vi "Initialize Menu Panel.vi"(8 "error in":errorcluster, 11 "Display State In":T1={"Numeric"=0.0, "Array of Button References"=[], "Space Between Menu Buttons"=0, "Number of Menu Buttons"=0, "Array of Button Names"=[], "Most Recent Vertical Position"=0, "This VI"=refnum, "Current Action"=enum."Not Moving", "Most Recent Distance Traveled"=0, "Method"=enum."Move Up", "Data In"=0}) -> (0 "error IO 2":errorcluster, 3 "Display State Out":T1={"Numeric"=0.0, "Array of Button References"=[], "Space Between Menu Buttons"=3, "Number of Menu Buttons"=6, "Array of Button Names"=[], "Most Recent Vertical Position"=0, "This VI"=refnum, "Current Action"=enum."Not Moving", "Most Recent Distance Traveled"=0, "Method"=enum."Resize", "Data In"=0} caption="State")   [LabVIEW 2011, in "Sliding Menu Library.lvlib" / "Sliding Menu XControl.xctl"]
uses:
  Sliding Menu xControl/Sliding Menu XControl.xctl
  Sliding Menu xControl/Sliding Menu State.ctl
  Menu Button Library/Menu Button xControl/Menu Button xControl.xctl
  Sliding Menu Type Definitions/Current User Action.ctl
  Sliding Menu xControl/Sliding Menu Methods.ctl
  Sliding Menu xControl/Sliding Menu Data.ctl
  <vilib>/Utility/miscctls.llb/LVPointTypeDef.ctl
  Sliding Menu Library.lvlib
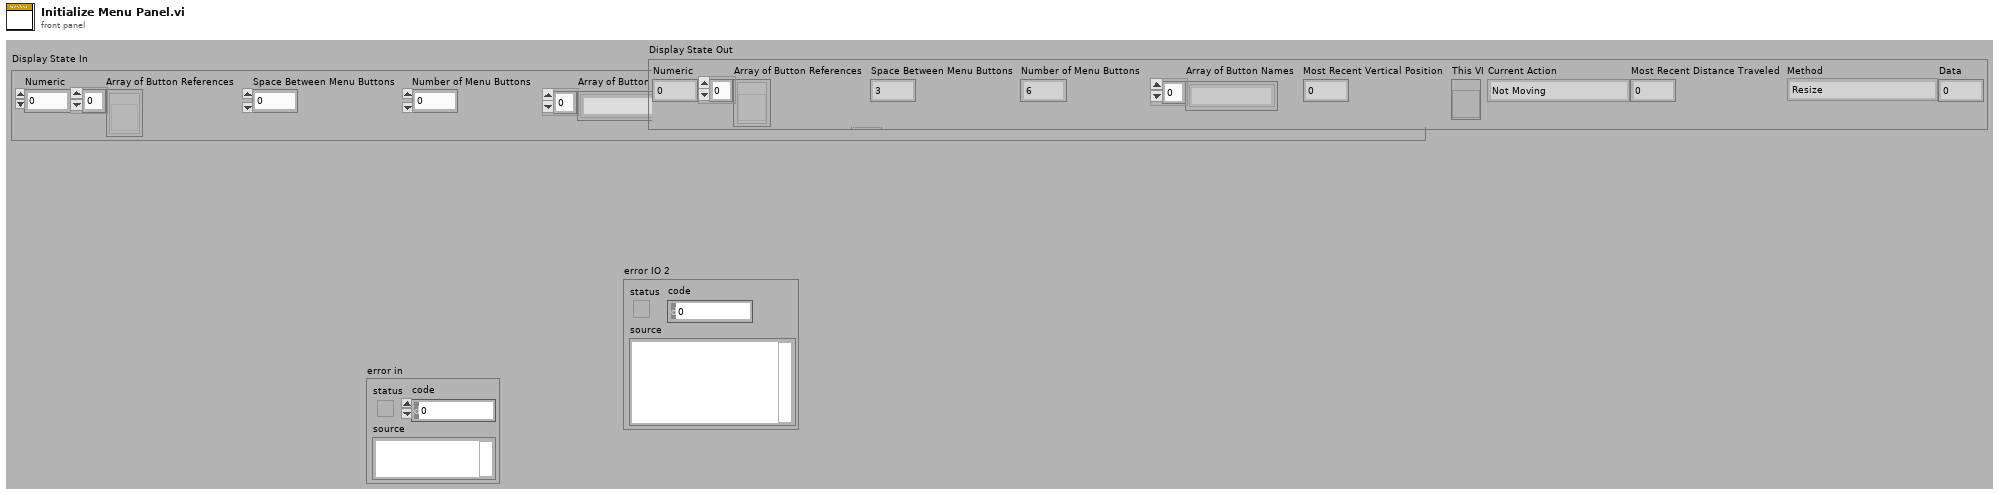
[diagram p1: front panel]
types:
  T1 = typedef "Sliding Menu Library.lvlib/Sliding Menu XControl.xctl/Sliding Menu State.ctl" = cluster{"Numeric":dbl, "Array of Button References":refnum<vi>[], "Space Between Menu Buttons":i32, "Number of Menu Buttons":i32, "Array of Button Names":string[], "Most Recent Vertical Position":i32, "This VI":refnum<vi>, "Current Action":T2, "Most Recent Distance Traveled":i32, "Method":T3, "Data In":T4}
  T2 = typedef "Sliding Menu Library.lvlib/Current User Action.ctl" = enum16{"Not Moving", "Mouse Down", "Mouse Up No Dragging", "Bounce Up Needed", "Bounce Down Needed", "Dragging", "Easing"}
  T3 = typedef "Sliding Menu Methods.ctl" = enum16{"Resize", "Move Up", "Move Down", "Move to 0"}
  T4 = typedef "Sliding Menu Library.lvlib/Sliding Menu XControl.xctl/Sliding Menu Data.ctl" = i32
  T5 = typedef "LVPointTypeDef.ctl" = cluster{"Horizontal":i16, "Vertical":i16}
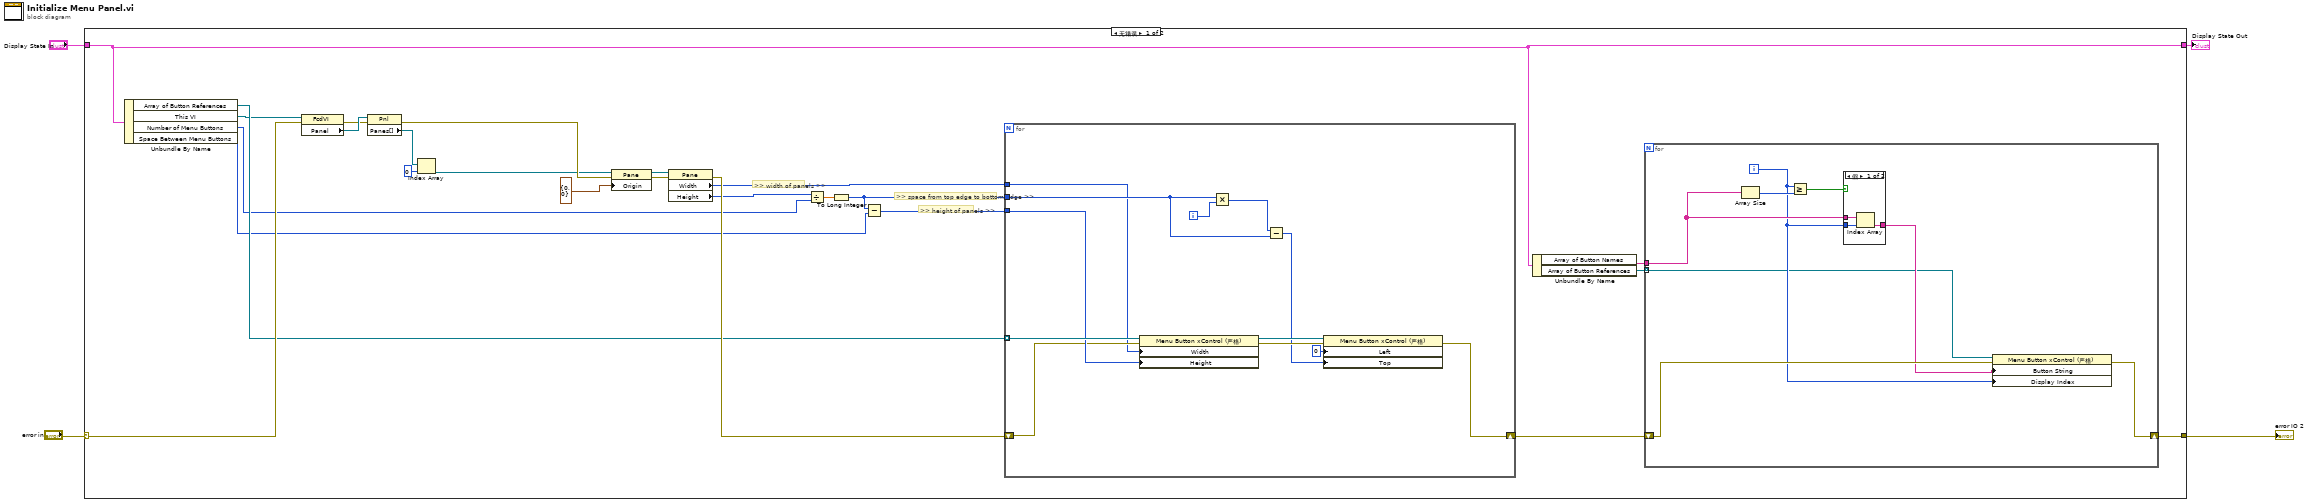
[diagram p0: block diagram]
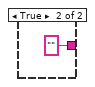
[diagram p2: hidden frame]
diagram:
  n1 = case shown="无错误" "error in" {
    selector: "error in" -> [w20 w54]
    tunnel: [w8 w54] -> w3
    tunnel: "Display State In" -> [w10 _]
    tunnel: [w10 _] -> w1
    frame No Error {
      # ">> height of panels >>"
      # ">> width of panels >>"
      # ">> space from top edge to bottom edge >>"
      n2 = Unbundle By Name(w10) -> ("Array of Button References"=w16:refnum<vi>[], "This VI"=w12:refnum<vi>, "Number of Menu Buttons"=w7:i32, "Space Between Menu Buttons"=w6:i32)
      n3 = property class="FcdVI"(reference=w12, error in=w20) -> (error out=w22:errorcluster, "Panel"=w23:refnum<vi>)  [unwired: 1 out]
      n4 = property class="Pnl"(reference=w23, error in=w22) -> (error out=w25:errorcluster, "Panes[]"=w15:refnum<vi>[])  [unwired: 1 out]
      n5 = Index Array(array=w15, index=0) -> (element=w14:refnum<vi>)
      n6 = property class="Pane"(reference=w14, error in=w25, "Origin"=T5 {"Horizontal"=0, "Vertical"=0}) -> (reference out=w18:refnum<vi>, error out=w26:errorcluster)
      n7 = property class="Pane"(reference=w18, error in=w26) -> (error out=w21:errorcluster, "Width"=w17:u32, "Height"=w19:u32)  [unwired: 1 out]
      n8 = Divide(x=w19, y=w7) -> (x/y=w27:dbl)
      n9 = To Long Integer(number=w27) -> (32bit integer=w28:i32)
      n10 = Subtract(x=w28, y=w6) -> (x-y=w29:i32)
      n11 = for {
        tunnel: w16 -> [w53] mode=indexing
        tunnel: w28 -> [w51]
        tunnel: w17 -> [w48]
        tunnel: w29 -> [w52]
        shift-right: [w50] -> w9
        shift-left: w21 -> [w49]
        i -> [w42]
        n12 = property class="Menu Button xControl (严格)"(reference=w53, error in=w49, "Width"=w48, "Height"=w52) -> (reference out=w47:refnum<vi>, error out=w46:errorcluster)
        n13 = Multiply(x=w51, y=w42) -> (x*y=w44:i32)
        n14 = Subtract(x=w44, y=w51) -> (x-y=w43:i32)
        n15 = property class="Menu Button xControl (严格)"(reference=w47, error in=w46, "Left"=0 ("Position:Left"), "Top"=w43) -> (error out=w50:errorcluster)  [unwired: 1 out]
      }
      n16 = Unbundle By Name(w10) -> ("Array of Button Names"=w11:string[], "Array of Button References"=w5:refnum<vi>[])
      n17 = for {
        shift-right: [w36] -> w8
        shift-left: w9 -> [w37]
        tunnel: w11 -> [w33]
        tunnel: w5 -> [w30] mode=indexing
        i -> [w31]
        n18 = Array Size(array=w33) -> (size(s)=w35:i32)
        n19 = Greater Or Equal?(x=w31, y=w35) -> (x >= y?=w34:bool)
        n20 = case shown="假" w34 {
          tunnel: [w40 "" ("String")] -> w32
          tunnel: w33 -> [w39 _]
          tunnel: w31 -> [w38 _]
          frame False {
            n21 = Index Array(array=w39, index=w38) -> (element=w40:string)
          }
          frame True {
          }
        }
        n22 = property class="Menu Button xControl (严格)"(reference=w30, error in=w37, "Button String"=w32, "Display Index"=w31) -> (error out=w36:errorcluster)  [unwired: 1 out]
      }
    }
    frame Error {
    }
  }
  "error IO 2" <- w3
  "Display State Out" <- w1
